vi "Initialize APSVG2.vi"(11 "Connection":string) -> (0 "error out":errorcluster, 1 "String":string, 2 "Serial number":string, 3 "VISA Refnum out":refnum<visa-resource-name>, 4 "trimmed string":string, 5 "Company":string, 6 "Checkbox":bool, 7 "FW version":string)   [LabVIEW 2024, in "THz source modeule.lvlib"]
uses:
  THz source modeule.lvlib
  <vilib>/Utility/error.llb/Trim Whitespace One-Sided.vi
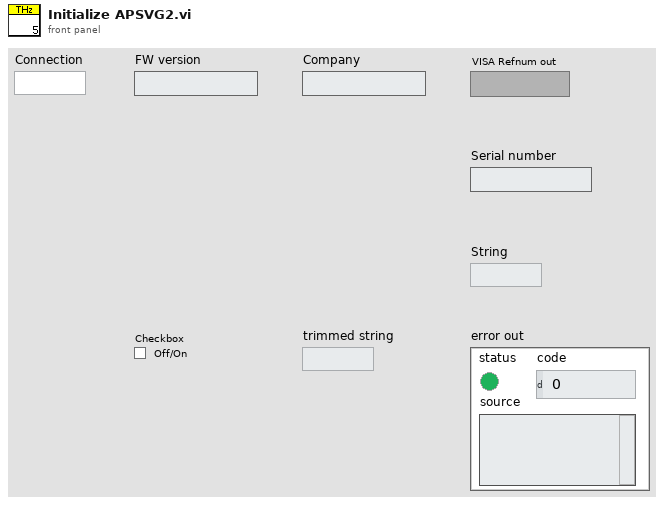
[diagram p1: front panel]
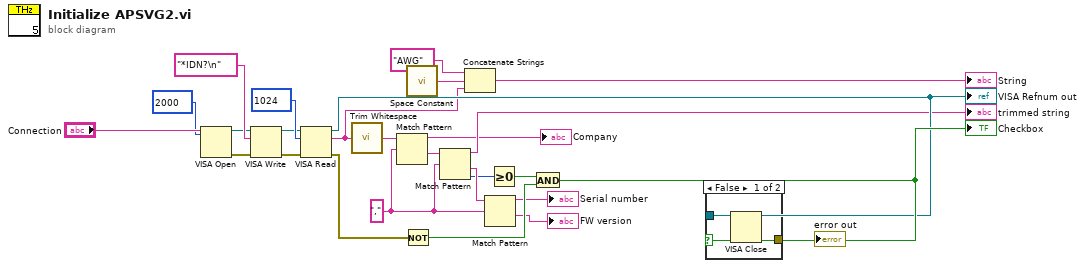
[diagram p0: block diagram]
diagram:
  w13 = "," ("regular expression")
  n1 = VISA Open(timeout (0)=2000, VISA resource name="Connection") -> (VISA resource name=w1:refnum<visa-resource-name>, error out=w2:errorcluster)  [unwired: 2 in, 1 out]
  n2 = VISA Write(VISA resource name=w1, write buffer="*IDN?\n", error in (no error)=w2) -> (VISA resource name out=w5:refnum<visa-resource-name>, error out=w4:errorcluster)  [unwired: 1 out]
  n3 = VISA Read(VISA resource name=w5, byte count=u32 1024, error in (no error)=w4) -> (VISA resource name out=w26:refnum<visa-resource-name>, read buffer=w21:string, error out=w23:errorcluster)  [unwired: 1 out]
  "VISA Refnum out" <- w26
  n4 = call <vilib>:"Trim Whitespace.vi"("string"=w21) -> ("trimmed string"=w11:string)  [unwired: 1 in]
  n5 = Match Pattern(string=w11, regular expression=w13) -> (before substring=→"Company":string, after substring=w8:string)  [unwired: 1 in, 2 out]
  n6 = Not(x=w23) -> (.not. x?=w25:bool)
  n7 = call <vilib>:"Space Constant.vi"() -> ("String"=w20:string)
  n8 = Match Pattern(string=w8, regular expression=w13) -> (before substring=→"trimmed string":string, after substring=w12:string, offset past match=w10:i32)  [unwired: 1 in, 1 out]
  n9 = Concatenate Strings("AWG" ("Description"), w20, w21) -> (→"String":string)
  n10 = Match Pattern(string=w12, regular expression=w13) -> (before substring=→"Serial number":string, after substring=→"FW version":string)  [unwired: 1 in, 2 out]
  n11 = Greater Or Equal To 0?(x=w10) -> (x >= 0?=w24:bool)
  n12 = And(x=w24, y=w25) -> (x .and. y?=w27:bool)
  "Checkbox" <- w27
  n13 = case shown="False" w27 {
    tunnel: [w29 _] -> w22
    tunnel: w26 -> [w28 _]
    frame False {
      n14 = VISA Close(VISA resource name=w28) -> (error out=w29:errorcluster)  [unwired: 1 in]
    }
    frame True {
    }
  }
  "error out" <- w22
